vi "RequestSVE.vi"() -> (6 "MirrorCoverMotor-00":T1, 7 "MirrorCoverMotor-04":T1, 8 "MirrorCoverMotor-01":T1, 9 "MirrorCoverMotor-05":T1, 10 "MirrorCoverMotor-02":T1, 11 "MirrorCoverMotor-06":T1, 12 "MirrorCoverMotor-03":T1, 13 "MirrorCoverMotor-07":T1, 14 "MirrorCoverControlScheme":T3, 15 "MirrorCoverControllerConfig":T2)   [LabVIEW 2015]
uses:
  <vilib>/lvdsc/NI_DSC.lvlib
panel:
  out "error out":errorcluster
  in  "error in (no error)":errorcluster
  in  "Variable List":i32(listbox)=-1
  in  "System Events":i32(listbox)=-1
  in  "Stop?":bool
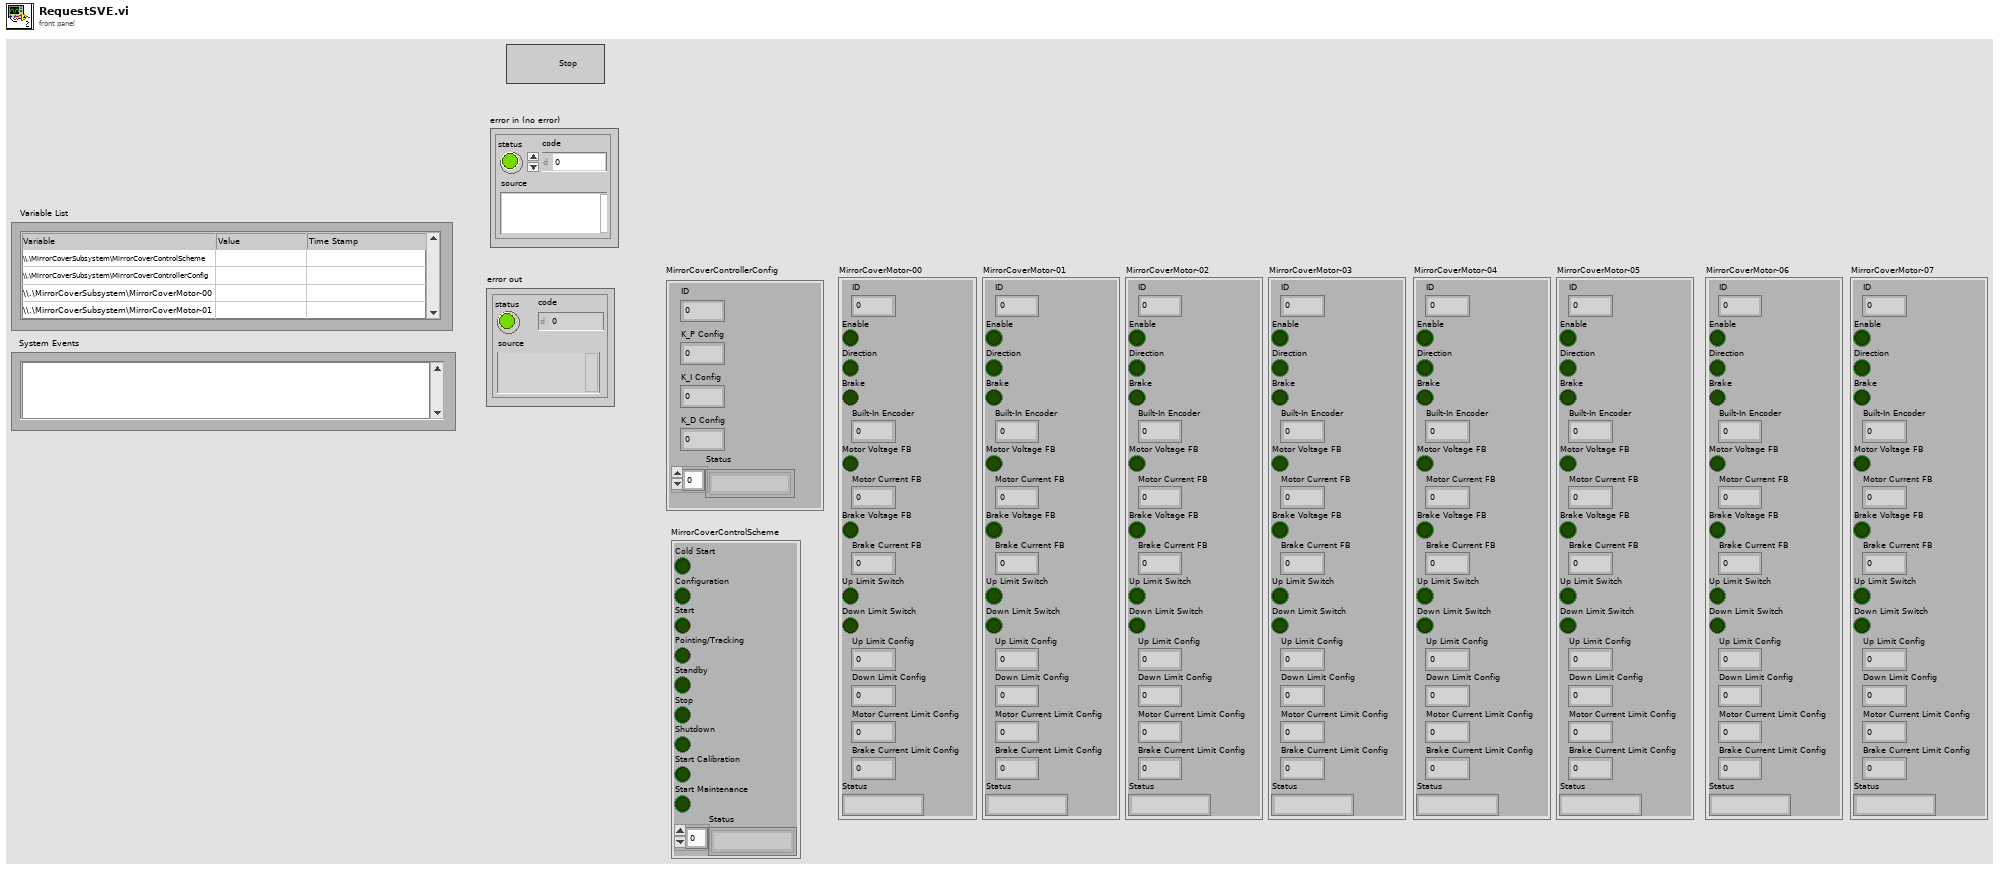
[diagram p1: front panel]
types:
  T1 = cluster{"ID":i32, "Enable":bool, "Direction":bool, "Brake":bool, "Built-In Encoder":u64, "Motor Voltage FB":bool, "Motor Current FB":u64, "Brake Voltage FB":bool, "Brake Current FB":u64, "Up Limit Switch":bool, "Down Limit Switch":bool, "Up Limit Config":u64, "Down Limit Config":u64, "Motor Current Limit Config":u64, "Brake Current Limit Config":u64, "Status":string}
  T2 = cluster{"ID":dbl, "K_P Config":dbl, "K_I Config":dbl, "K_D Config":dbl, "Status":string[]}
  T3 = cluster{"Cold Start":bool, "Configuration":bool, "Start":bool, "Pointing/Tracking":bool, "Standby":bool, "Stop":bool, "Shutdown":bool, "Start Calibration":bool, "Start Maintenance":bool, "Status":string[]}
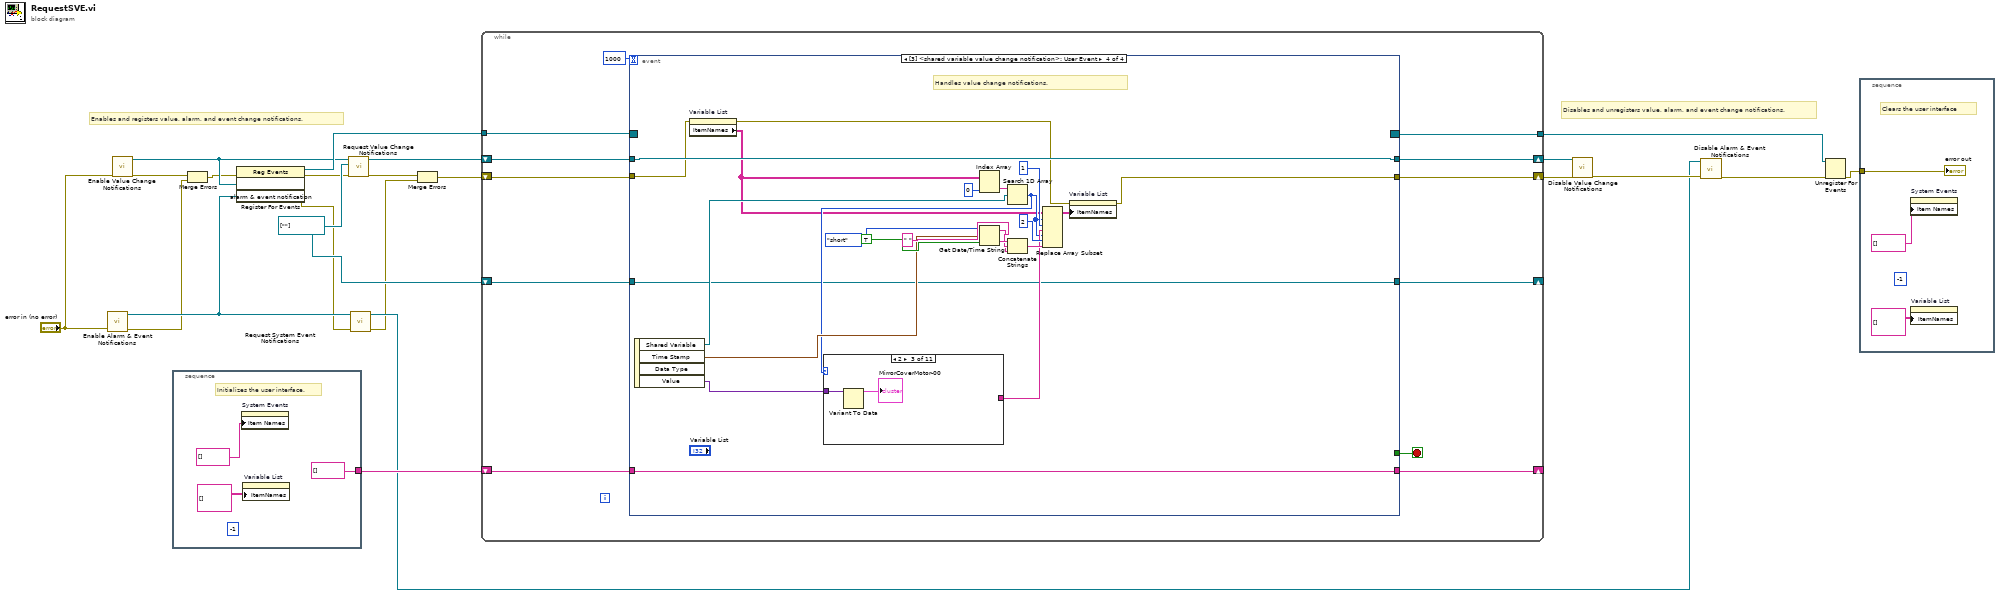
[diagram p0: block diagram]
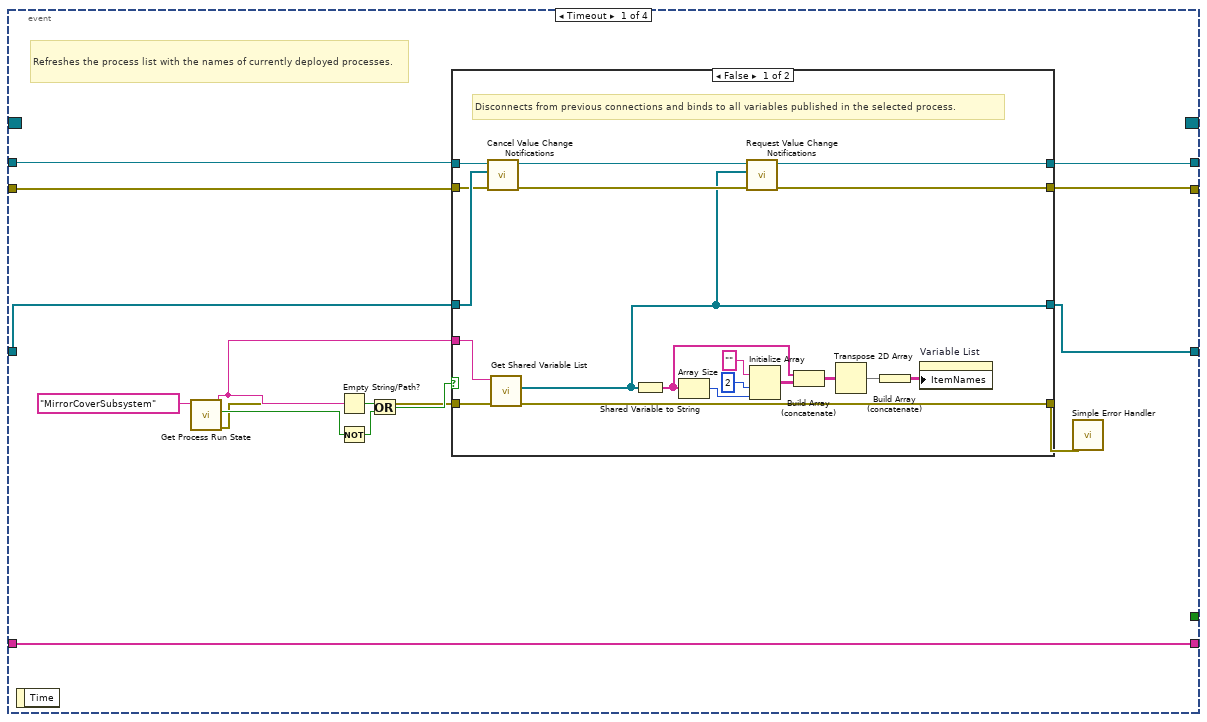
[diagram p2: hidden frame]
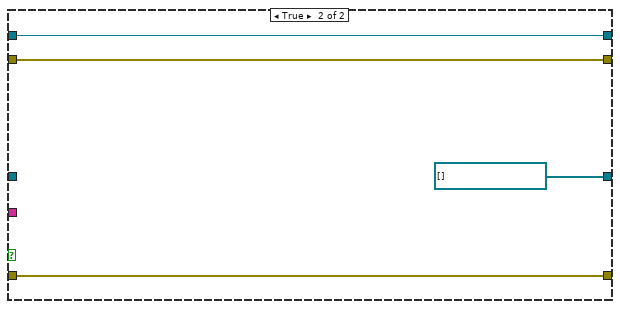
[diagram p3: hidden frame]
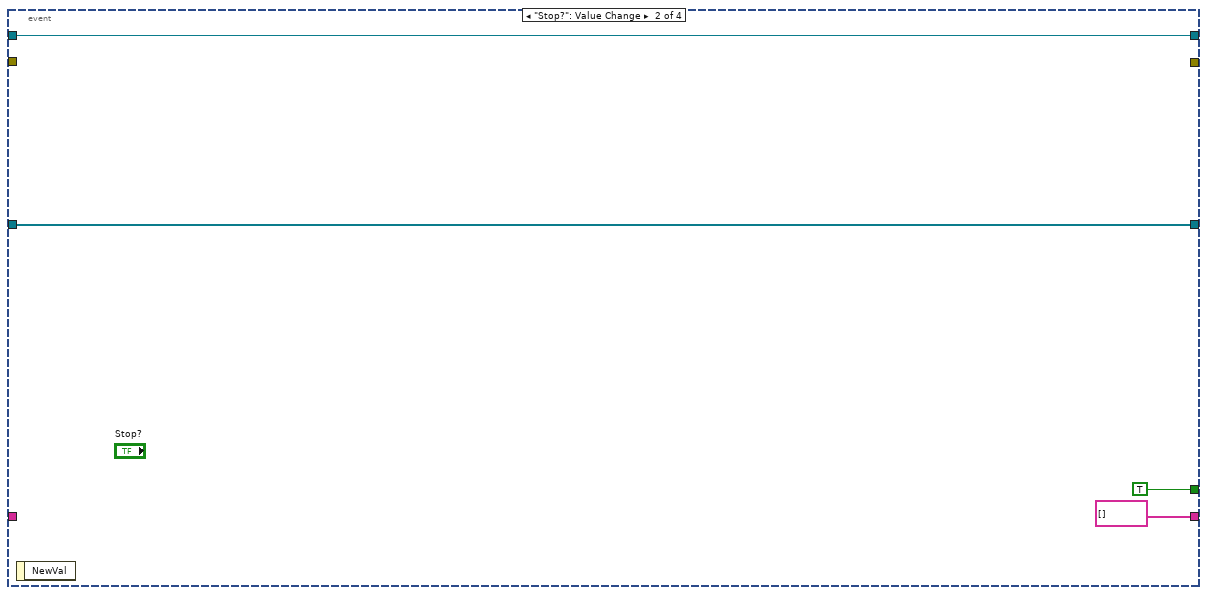
[diagram p4: hidden frame]
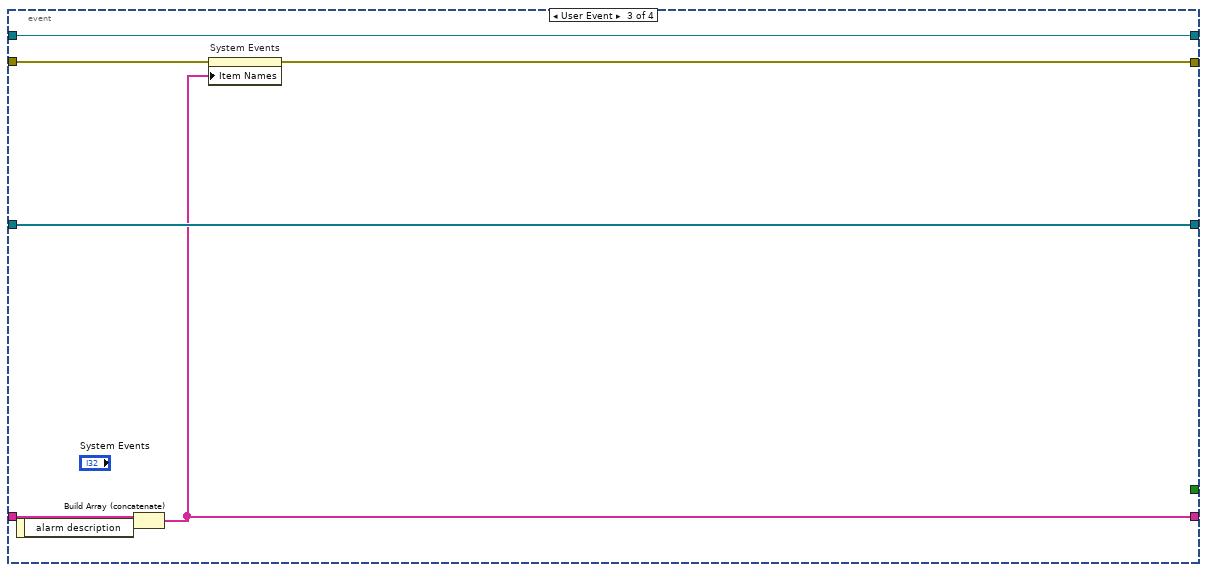
[diagram p5: hidden frame]
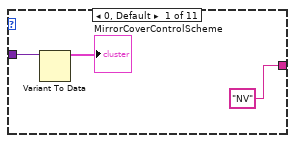
[diagram p6: hidden frame]
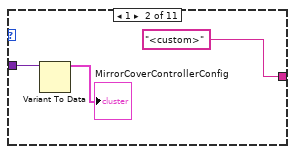
[diagram p7: hidden frame]
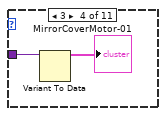
[diagram p8: hidden frame]
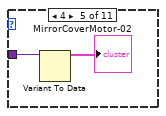
[diagram p9: hidden frame]
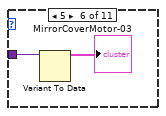
[diagram p10: hidden frame]
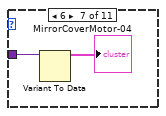
[diagram p11: hidden frame]
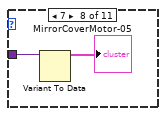
[diagram p12: hidden frame]
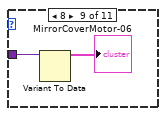
[diagram p13: hidden frame]
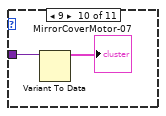
[diagram p14: hidden frame]
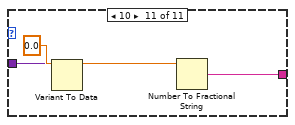
[diagram p15: hidden frame]
diagram:
  w20 = refnum<k21>[] [""] ("shared variables")
  # "Disables and unregisters value, alarm, and event change notifications."
  # "Enables and registers value, alarm, and event change notifications."
  n1 = call <vilib>:"Enable Alarm & Event Notifications.vi"("error in (no error)"="error in (no error)") -> ("error out"=w5:errorcluster, "alarm & event notification"=w8:refnum<user-event>)  [unwired: 9 out]
  n2 = call <vilib>:"Enable Value Change Notifications.vi"("error in (no error)"="error in (no error)") -> ("error out"=w7:errorcluster, "shared variable value change notification"=w9:refnum<user-event>)  [unwired: 9 out]
  n3 = stacked-sequence {
    tunnel: [string[] []] -> w17
    frame #0 {
      (unwired) -1 ("Process List")
      # "Initializes the user interface."
      n4 = property on="System Events" class="LstBox (strict)"("Item Names"=string[] []) -> ()  [unwired: 2 in, 2 out]
      n5 = property on="Variable List" class="MCListbox (strict)"("ItemNames"=string[][] [] ("Item Names")) -> ()  [unwired: 2 in, 2 out]
    }
  }
  n6 = Merge Errors(w7, w5) -> (w6:errorcluster)
  n7 = register-events(error in=w6, w9, w8) -> (reference out=w21:refnum<event-registration>, error out=w4:errorcluster)  [unwired: 1 in]
  n8 = call <vilib>:"Request Value Change Notifications.vi"("error in (no error)"=w4, "shared variables"=w20, "notification refnum"=w9) -> ("error out"=w3:errorcluster, "shared variable value change notification"=w12:refnum<user-event>)  [unwired: 1 in, 6 out]
  n9 = call <vilib>:"Request System Event Notifications.vi"("error in (no error)"=w4, "notification refnum"=w8) -> ("error out"=w2:errorcluster, "alarm & event notification"=w14:refnum<user-event>)  [unwired: 1 in, 7 out]
  n10 = Merge Errors(w3, w2) -> (w1:errorcluster)
  n11 = while {
    tunnel: w21 -> [w35]
    shift-right: [w33] -> _
    shift-left: w17 -> [w34]
    shift-right: [w25] -> _
    shift-left: w20 -> [w30]
    shift-right: [w29] -> w19
    shift-left: w12 -> [w31]
    tunnel: [w28] -> w11
    shift-right: [w27] -> w13
    shift-left: w1 -> [w26]
    stop <- w36 stop-if-true
    n12 = event shown="[3] <shared variable value change notification>: User Event" {
      selector: w35 -> [_ _ _ _]
      dyn-events: [_ _ _ _] -> w28
      timeout: 1000 -> [_ _ _ _]
      tunnel: [_ TRUE ("Stop?") _ _] -> w36
      tunnel: w31 -> [w47 w76 w82 w100]
      tunnel: w34 -> [w51 _ w85 w108]
      tunnel: [w51 string[] [] w81 w108] -> w33
      tunnel: w30 -> [w50 w77 w83 w86]
      tunnel: [_ w77 w83 w86] -> w25
      tunnel: [w46 w76 w82 w100] -> w29
      tunnel: w26 -> [w49 _ w79 w88]
      tunnel: [w48 _ w80 w98] -> w27
      tunnel: [w37 _ _ _] -> _
      event Timeout {
        # "Refreshes the process list with the names of currently deployed processes."
        n13 = event-data() -> ()  [unwired: 2 out]
        n14 = call <vilib>:"Get Process Run State.vi"("process name"="MirrorCoverSubsystem") -> ("error out"=w39:errorcluster, "exists?"=w40:bool, "process name out"=w41:string)  [unwired: 1 in, 7 out]
        n15 = Empty String/Path?(string/path=w41) -> (empty?=w44:bool)
        n16 = Not(x=w40) -> (.not. x?=w45:bool)
        n17 = Or(x=w44, y=w45) -> (x .or. y?=w43:bool)
        n18 = case shown="False" w43 {
          tunnel: w41 -> [w70 _]
          tunnel: w50 -> [w67 _]
          tunnel: w47 -> [w66 w73]
          tunnel: [w59 w73] -> w46
          tunnel: [w55 refnum<k21>[] [] ("shared variables")] -> w37
          tunnel: w39 -> [w56 w71]
          tunnel: w49 -> [w54 w72]
          tunnel: [w53 w72] -> w48
          tunnel: [w52 w71] -> w38
          frame False {
            # "Disconnects from previous connections and binds to all variables published in the selected process."
            n19 = call <vilib>:"Cancel Value Change Notifications.vi"("error in (no error)"=w54, "shared variables"=w67, "notification refnum"=w66) -> ("error out"=w68:errorcluster, "shared variable value change notification"=w69:refnum<user-event>)  [unwired: 7 out]
            n20 = call <vilib>:"Get Shared Variable List.vi"("error in (no error)"=w56, "process name"=w70) -> ("error out"=w52:errorcluster, "shared variables"=w55:refnum<k21>[])  [unwired: 8 out]
            n21 = Shared Variable to String(1:w55) -> (0:w58:string[])
            n22 = Array Size(array=w58) -> (size(s)=w60:i32)
            n23 = call <vilib>:"Request Value Change Notifications.vi"("error in (no error)"=w68, "shared variables"=w55, "notification refnum"=w69) -> ("error out"=w53:errorcluster, "shared variable value change notification"=w59:refnum<user-event>)  [unwired: 1 in, 6 out]
            n24 = Initialize Array("", 2 ("dimension size"), w60) -> (w62:string[][])
            n25 = Build Array (concatenate)(w58, w62) -> (w61:string[][])
            n26 = Transpose 2D Array(2D array=w61) -> (transposed array=w65:string[][])
            n27 = Build Array (concatenate)(w65) -> (w64:string[][])
            n28 = property on="Variable List" class="MCListbox (strict)"("ItemNames"=w64) -> ()  [unwired: 2 in, 2 out]
          }
          frame True {
          }
        }
        n29 = call <vilib>:"Simple Error Handler.vi"("error in (no error)"=w38) -> ()  [unwired: 4 in, 5 out]
      }
      event "Stop?": Value Change {
        n30 = event-data() -> ()  [unwired: 2 out]
      }
      event User Event {
        n31 = event-data() -> ("alarm description"=w84:string)  [unwired: 1 out]
        n32 = Build Array (concatenate)(w85, w84) -> (w81:string[])
        n33 = property on="System Events" class="LstBox (strict)"(error in=w79, "Item Names"=w81) -> (error out=w80:errorcluster)  [unwired: 1 in, 1 out]
      }
      event User Event {
        # "Handles value change notifications."
        n34 = event-data() -> ("Shared Variable"=w92:refnum<k21>, "Time Stamp"=w99:timestamp, "Value"=w90:variant)  [unwired: 2 out]
        n35 = property on="Variable List" class="MCListbox (strict)"(error in=w88) -> (error out=w95:errorcluster, "ItemNames"=w87:string[][])  [unwired: 1 in, 1 out]
        n36 = Index Array(array=w87, index (col)=0 ("disabled index (col)")) -> (element=w93:string[])  [unwired: 1 in]
        n37 = Get Date/Time String(date format (0)=enum16{"short", "long", "abbreviated"}."short", seconds (now)=w99, want seconds? (F)=TRUE) -> (date string=w97:string, time string=w106:string)
        n38 = Search 1D Array(1D array=w93, element=w92) -> (index of element=w89:i32)  [unwired: 1 out]
        n39 = case shown="2" w89 {
          tunnel: w90 -> [w109 w113 w116 w117 w119 w121 w123 w125 w127 w129 w131]
          tunnel: ["NV" "<custom>" _ _ _ _ _ _ _ _ w132] -> w91
          frame 0, Default {
            n40 = Variant To Data(Variant=w109) -> (data=→"MirrorCoverControlScheme":T3)  [unwired: 2 in, 1 out]
          }
          frame 1 {
            n41 = Variant To Data(Variant=w113) -> (data=→"MirrorCoverControllerConfig":T2)  [unwired: 2 in, 1 out]
          }
          frame 2 {
            n42 = Variant To Data(Variant=w116) -> (data=→"MirrorCoverMotor-00":T1)  [unwired: 2 in, 1 out]
          }
          frame 3 {
            n43 = Variant To Data(Variant=w117) -> (data=→"MirrorCoverMotor-01":T1)  [unwired: 2 in, 1 out]
          }
          frame 4 {
            n44 = Variant To Data(Variant=w119) -> (data=→"MirrorCoverMotor-02":T1)  [unwired: 2 in, 1 out]
          }
          frame 5 {
            n45 = Variant To Data(Variant=w121) -> (data=→"MirrorCoverMotor-03":T1)  [unwired: 2 in, 1 out]
          }
          frame 6 {
            n46 = Variant To Data(Variant=w123) -> (data=→"MirrorCoverMotor-04":T1)  [unwired: 2 in, 1 out]
          }
          frame 7 {
            n47 = Variant To Data(Variant=w125) -> (data=→"MirrorCoverMotor-05":T1)  [unwired: 2 in, 1 out]
          }
          frame 8 {
            n48 = Variant To Data(Variant=w127) -> (data=→"MirrorCoverMotor-06":T1)  [unwired: 2 in, 1 out]
          }
          frame 9 {
            n49 = Variant To Data(Variant=w129) -> (data=→"MirrorCoverMotor-07":T1)  [unwired: 2 in, 1 out]
          }
          frame 10 {
            n50 = Variant To Data(type=sgl 0.0 ("disabled index (col)"), Variant=w131) -> (data=w133:sgl)  [unwired: 1 in, 1 out]
            n51 = Number To Fractional String(number=w133) -> (F-format string=w132:string)  [unwired: 3 out]
          }
        }
        n52 = Concatenate Strings(w106, " " ("string"), w97) -> (w103:string)
        n53 = Replace Array Subset(array=w87, new element #1=w91, index (row) #1=w89, index (col) #1=1 ("disabled index (row)"), new element #2=w103, index (row) #2=w89, index (col) #2=2 ("index (col)")) -> (w96:string[][])
        n54 = property on="Variable List" class="MCListbox (strict)"(error in=w95, "ItemNames"=w96) -> (error out=w98:errorcluster)  [unwired: 1 in, 1 out]
      }
    }
  }
  n55 = call <vilib>:"Disable Value Change Notifications.vi"("error in (no error)"=w13, "notification refnum"=w19) -> ("error out"=w16:errorcluster)  [unwired: 9 out]
  n56 = call <vilib>:"Disable Alarm & Event Notifications.vi"("error in (no error)"=w16, "notification refnum"=w14) -> ("error out"=w15:errorcluster)  [unwired: 9 in]
  n57 = Unregister For Events(event registration refnum=w11, error in=w15) -> (error out=w18:errorcluster)
  n58 = stacked-sequence {
    tunnel: w18 -> [w135]
    frame #0 {
      (unwired) -1 ("Process List")
      # "Clears the user interface"
      n59 = property on="System Events" class="LstBox (strict)"("Item Names"=string[] []) -> ()  [unwired: 2 in, 2 out]
      n60 = property on="Variable List" class="MCListbox (strict)"("ItemNames"=string[][] [] ("Item Names")) -> ()  [unwired: 2 in, 2 out]
      "error out" <- w135
    }
  }
